vi "Teleop.vi"(10 "Match Info":T1={"Autonomous Elapsed Seconds"=0.0, "TeleOp Elapsed Seconds"=0.0, "Disabled Elapsed Seconds"=0.0, "Visited Autonomous"=FALSE, "Visited TeleOp"=FALSE, "Visited Disabled"=FALSE, "Autonomous Settings"={"Autonomous Style"=enum."Independent", "VI Refnum"=refnum}}, 11 "Call Context":T2) -> ()   [LabVIEW 2017]
doc: "This VI is called for each TeleOp packet received from the DS where the robot is not disabled. It is often used to read from the joysticks and update I/O or to update setpoints for timed control loops. It should complete and return within 20 milliseconds or it may miss DS packets."
uses:
  <vilib>/Rock Robotics/WPI/DriverStation/WPI_DriverStationDerivedRobotMode.ctl
  <vilib>/Rock Robotics/WPI/DriverStation/WPI_DriverStationMatch Info.ctl
  <vilib>/Rock Robotics/WPI/Solenoid/WPI_SolenoidValue.ctl
  <vilib>/Rock Robotics/WPI/ThirdParty/Sensors/navX/_TypeDefs/FRIC_navX_DeviceNumbersTypeDef.ctl
  <vilib>/Rock Robotics/WPI/Utilities/WPI_GetSetVariantRefNum.vi
  Robot Global Data.vi
  <vilib>/Rock Robotics/WPI/Solenoid/WPI_SolenoidSetEnum.vi
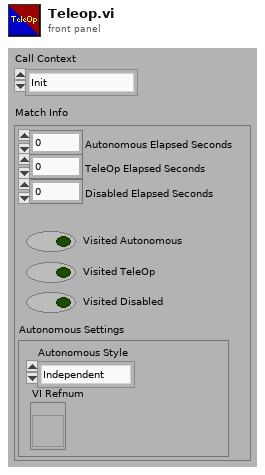
[diagram p1: front panel]
types:
  T1 = typedef "WPI_DriverStationMatch Info.ctl" = cluster{"Autonomous Elapsed Seconds":dbl, "TeleOp Elapsed Seconds":dbl, "Disabled Elapsed Seconds":dbl, "Visited Autonomous":bool, "Visited TeleOp":bool, "Visited Disabled":bool, "Autonomous Settings":cluster{"Autonomous Style":enum16{"Iterative", "Independent"}, "VI Refnum":refnum<vi>}}
  T2 = typedef "WPI_DriverStationDerivedRobotMode.ctl" = enum16{"Init", "Execute", "Stop"}
  T3 = enum16{"Manual", "Turn For Angle", "Drive For Distance", "Motion Profile"}
  T4 = typedef "WPI_SolenoidValue.ctl" = enum16{"Off", "On", "Forward", "Reverse"}
  T5 = typedef "WPI_JoystickDevRef.ctl" = cluster{"Device":T6}
  T6 = typedef "WPI_JoystickDeviceEnum.ctl" = enum16{"USB 0", "USB 1", "USB 2", "USB 3", "USB 4", "USB 5"}
  T7 = typedef "WPI_SolenoidDevRef.ctl" = cluster{"DevStatus":errorcluster, "Pneumatics Control Module":u8, "Forward Solenoid Channel":T8, "Reverse Solenoid Channel":T8}
  T8 = typedef "WPI_SolenoidChannel.ctl" = enum8{"Solenoid 0", "Solenoid 1", "Solenoid 2", "Solenoid 3", "Solenoid 4", "Solenoid 5", "Solenoid 6", "Solenoid 7", "Invalid"}
  T9 = typedef "FRIC_navX_DeviceNumbersTypeDef.ctl" = enum16{"Dev0", "Dev1", "Dev2", "Dev3"}
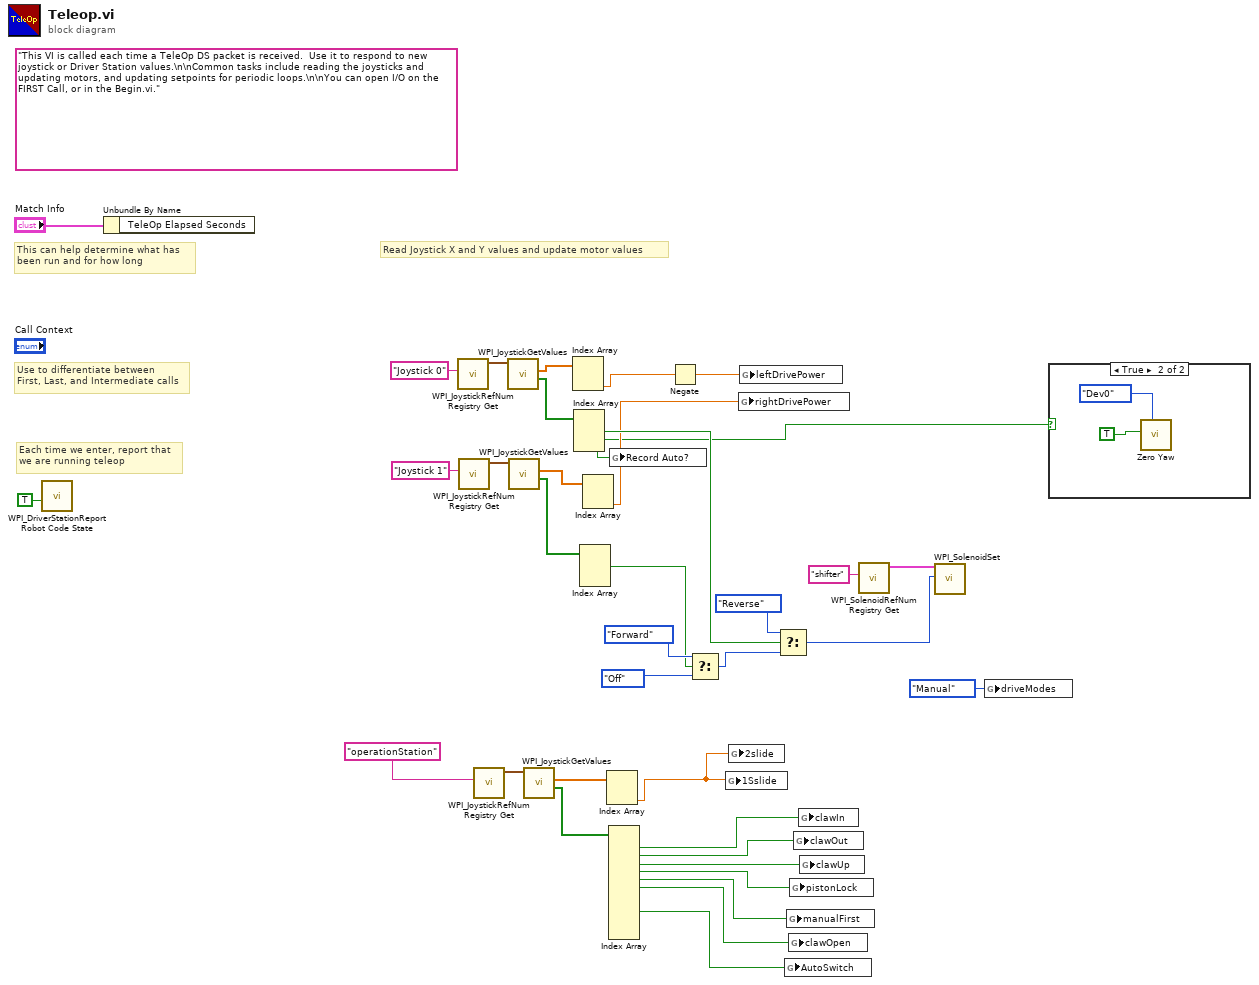
[diagram p0: block diagram]
diagram:
  (unwired) "This VI is called each time a TeleOp DS packet is received.  Use it to respond to new joystick or Driver Station values.\n\nCommon tasks include reading the joysticks and updating motors, and updating setpoints for periodic loops.\n\nYou can open I/O on the FIRST Call, or in the Begin.vi."
  # "Each time we enter, report that\nwe are running teleop"
  # "Use to differentiate between\nFirst, Last, and Intermediate calls"
  # "This can help determine what has\nbeen run and for how long"
  # "Read Joystick X and Y values and update motor values"
  n1 = call <vilib>:"WPI_DriverStationReport Robot Code State.vi"("TeleOp"=TRUE ("Autonomous")) -> ()  [unwired: 10 in, 1 out]
  n2 = Unbundle By Name("Match Info") -> ()  [unwired: 1 out]
  n3 = call <vilib>:"WPI_JoystickRefNum Registry Get.vi"("refnum name"="Joystick 0") -> ("JoystickDevRef"=w20:T5)  [unwired: 1 in, 9 out]
  n4 = call <vilib>:"WPI_JoystickRefNum Registry Get.vi"("refnum name"="Joystick 1") -> ("JoystickDevRef"=w19:T5)  [unwired: 1 in, 9 out]
  n5 = call <vilib>:"WPI_JoystickRefNum Registry Get.vi"("refnum name"="operationStation") -> ("JoystickDevRef"=w27:T5)  [unwired: 1 in, 9 out]
  n6 = call <vilib>:"WPI_JoystickGetValues.vi"("JoystickDevRef"=w20) -> ("Buttons"=w14:bool[], "Axes"=w12:dbl[])  [unwired: 6 in, 3 out]
  n7 = call <vilib>:"WPI_JoystickGetValues.vi"("JoystickDevRef"=w19) -> ("Buttons"=w16:bool[], "Axes"=w11:dbl[])  [unwired: 6 in, 3 out]
  n8 = call <vilib>:"WPI_JoystickGetValues.vi"("JoystickDevRef"=w27) -> ("Buttons"=w25:bool[], "Axes"=w26:dbl[])  [unwired: 6 in, 3 out]
  n9 = Index Array(array=w12) -> (element #2=w9:dbl)  [unwired: 2 in, 1 out]
  n10 = Index Array(array=w14) -> (element #1=w13:bool, element #2=w7:bool, element #3=w4:bool)  [unwired: 3 in]
  n11 = Index Array(array=w16) -> (element #1=w15:bool)  [unwired: 3 in, 2 out]
  n12 = Index Array(array=w11) -> (element #2=w10:dbl)  [unwired: 2 in, 1 out]
  n13 = Index Array(array=w26) -> (element #2=w24:dbl)  [unwired: 2 in, 1 out]
  n14 = Index Array(array=w25) -> (element #1=w23:bool, element #2=w22:bool, element #3=w3:bool, element #4=w6:bool, element #5=w21:bool, element #6=w2:bool, element #9=w1:bool)  [unwired: 12 in, 5 out]
  n15 = global write "Robot Global Data.vi" "Record Auto?"(w4) -> ()
  n16 = Negate(x=w9) -> (-x=w8:dbl)
  n17 = Select(t=WPI_SolenoidValue."Forward", s=w15, f=WPI_SolenoidValue."Off" ("Value")) -> (s? t:f=w34:T4)
  n18 = global write "Robot Global Data.vi" "1Sslide"(w24) -> ()
  n19 = global write "Robot Global Data.vi" "2slide"(w24) -> ()
  n20 = global write "Robot Global Data.vi" "rightDrivePower"(w10) -> ()
  n21 = global write "Robot Global Data.vi" "leftDrivePower"(w8) -> ()
  n22 = Select(t=WPI_SolenoidValue."Reverse", s=w13, f=w34) -> (s? t:f=w30:T4)
  n23 = global write "Robot Global Data.vi" "AutoSwitch"(w1) -> ()
  n24 = global write "Robot Global Data.vi" "manualFirst"(w21) -> ()
  n25 = global write "Robot Global Data.vi" "clawOpen"(w2) -> ()
  n26 = global write "Robot Global Data.vi" "pistonLock"(w6) -> ()
  n27 = global write "Robot Global Data.vi" "clawOut"(w22) -> ()
  n28 = global write "Robot Global Data.vi" "clawIn"(w23) -> ()
  n29 = global write "Robot Global Data.vi" "clawUp"(w3) -> ()
  n30 = call <vilib>:"WPI_SolenoidRefNum Registry Get.vi"("refnum name"="shifter") -> ("SolenoidDevRef"=w29:T7)  [unwired: 9 in, 1 out]
  n31 = call-poly <vilib>:"WPI_SolenoidSet.vi"("Value"=w30, "SolenoidDevRef"=w29) -> ()  [unwired: 8 in, 2 out]
  n32 = global write "Robot Global Data.vi" "driveModes"(T3."Manual" ("driveModes")) -> ()
  n33 = case shown="True" w7 {
    frame False {
    }
    frame True {
      n34 = call <vilib>:"Zero Yaw.vi"("Device Number"=FRIC_navX_DeviceNumbersTypeDef."Dev0", "Zero"=TRUE) -> ()  [unwired: 10 in]
    }
  }
